vi "Load File Image Source.vi"(8 "error in":errorcluster, 11 "Image In":T1) -> (0 "error out":errorcluster, 2 "Image Dst Out":T1)   [LabVIEW 2015]
uses:
  <vilib>/vision/Image Controls.llb/IMAQ Image.ctl
panel:
  in  "Image Dst":T1
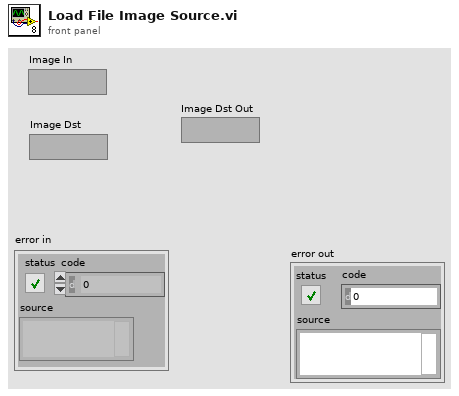
[diagram p1: front panel]
types:
  T1 = typedef "IMAQ Image.ctl" = refnum<image>
  T2 = typedef "Image Type" = u32
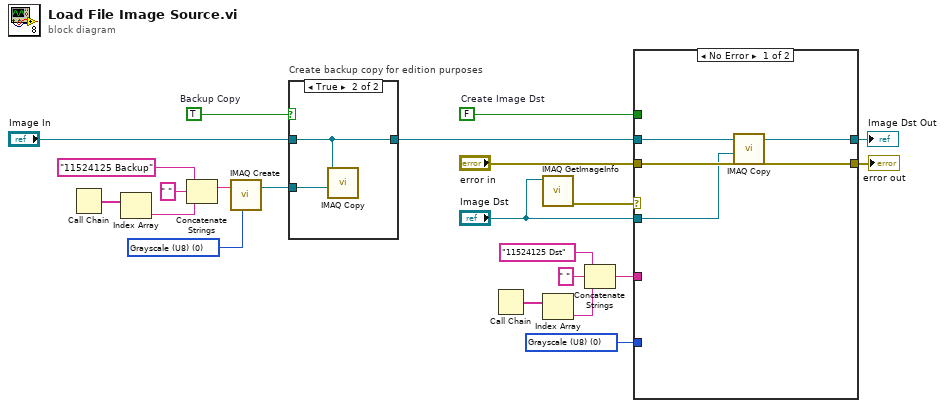
[diagram p0: block diagram]
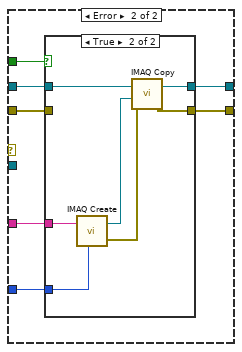
[diagram p2: hidden frame]
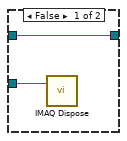
[diagram p4: hidden frame]
diagram:
  w3 = T2 0 items=["Grayscale (U8)", "Grayscale (I16)", "Grayscale (SGL)", "Complex (CSG)", "RGB (U32)", "HSL (U32)", "RGB (U64)", "Grayscale (U16)"] ("Image Dst Type")
  w4 = T2 0 items=["Grayscale (U8)", "Grayscale (I16)", "Grayscale (SGL)", "Complex (CSG)", "RGB (U32)", "HSL (U32)", "RGB (U64)", "Grayscale (U16)"] ("Image Type")
  w22 = TRUE  # Backup Copy
  w16 = FALSE  # Create Image Dst
  n1 = Call Chain() -> (call chain=w10:string[])
  n2 = Index Array(array=w10) -> (element=w9:string)  [unwired: 1 in]
  n3 = Concatenate Strings("11524125 Backup" ("Backup Image Name"), " ", w9) -> (w6:string)
  n4 = call "IMAQ Create"("Image Name"=w6, "Image Type"=w4) -> ("New Image"=w5:T1)  [unwired: 2 in, 2 out]
  n5 = case "Create backup copy for edition purposes" shown="True" w22 {
    tunnel: [w24 w26] -> w18
    tunnel: "Image In" -> [w24 w26]
    tunnel: w5 -> [w23 w25]
    frame False {
      n6 = call "IMAQ Dispose"("Image"=w23) -> ()  [unwired: 2 in, 4 out]
    }
    frame True {
      n7 = call "IMAQ Copy"("Image Dst"=w25, "Image Src"=w26) -> ()  [unwired: 1 in, 5 out]
    }
  }
  n8 = Call Chain() -> (call chain=w15:string[])
  n9 = call "IMAQ GetImageInfo"("Image"="Image Dst") -> ("error out"=w20:errorcluster)  [unwired: 1 in, 9 out]
  n10 = Index Array(array=w15) -> (element=w13:string)  [unwired: 1 in]
  n11 = Concatenate Strings("11524125 Dst" ("Image Dst Name"), " ", w13) -> (w11:string)
  n12 = case shown="No Error" w20 {
    tunnel: [w31 w35] -> w2
    tunnel: [w30 w34] -> w1
    tunnel: w18 -> [w29 w36]
    tunnel: "error in" -> [w28 w32]
    tunnel: "Image Dst" -> [w27 _]
    tunnel: w11 -> [_ w38]
    tunnel: w3 -> [_ w37]
    tunnel: w16 -> [_ w33]
    frame No Error {
      n13 = call "IMAQ Copy"("error in (no error)"=w28, "Image Dst"=w27, "Image Src"=w29) -> ("error out"=w30:errorcluster, "Image Dst Out"=w31:T1)  [unwired: 3 out]
    }
    frame Error {
      n14 = case shown="True" w33 {
        tunnel: w38 -> [_ w47]
        tunnel: w37 -> [_ w46]
        tunnel: w36 -> [w40 w44]
        tunnel: [w40 w43] -> w35
        tunnel: [w39 w42] -> w34
        tunnel: w32 -> [w39 _]
        frame False {
        }
        frame True {
          n15 = call "IMAQ Create"("Image Name"=w47, "Image Type"=w46) -> ("New Image"=w45:T1, "error out"=w41:errorcluster)  [unwired: 2 in, 1 out]
          n16 = call "IMAQ Copy"("error in (no error)"=w41, "Image Dst"=w45, "Image Src"=w44) -> ("error out"=w42:errorcluster, "Image Dst Out"=w43:T1)  [unwired: 3 out]
        }
      }
    }
  }
  "Image Dst Out" <- w2
  "error out" <- w1
